vi "ImageFile_GetFolderImageFiles.vi"(8 "error in (no error)":errorcluster, 11 "File Path":path) -> (0 "error out":errorcluster, 3 "Folder Image Files":path[](array[path]))   [LabVIEW 2019]
panel:
  out "index of element":i32
  out "filenames":string[](array[string])
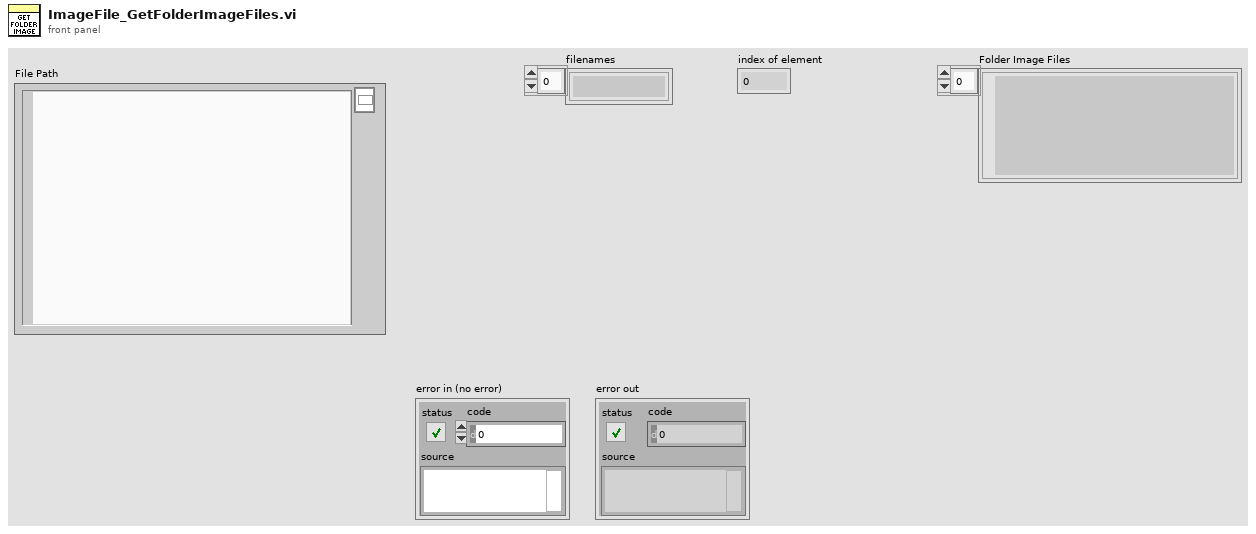
[diagram p1: front panel]
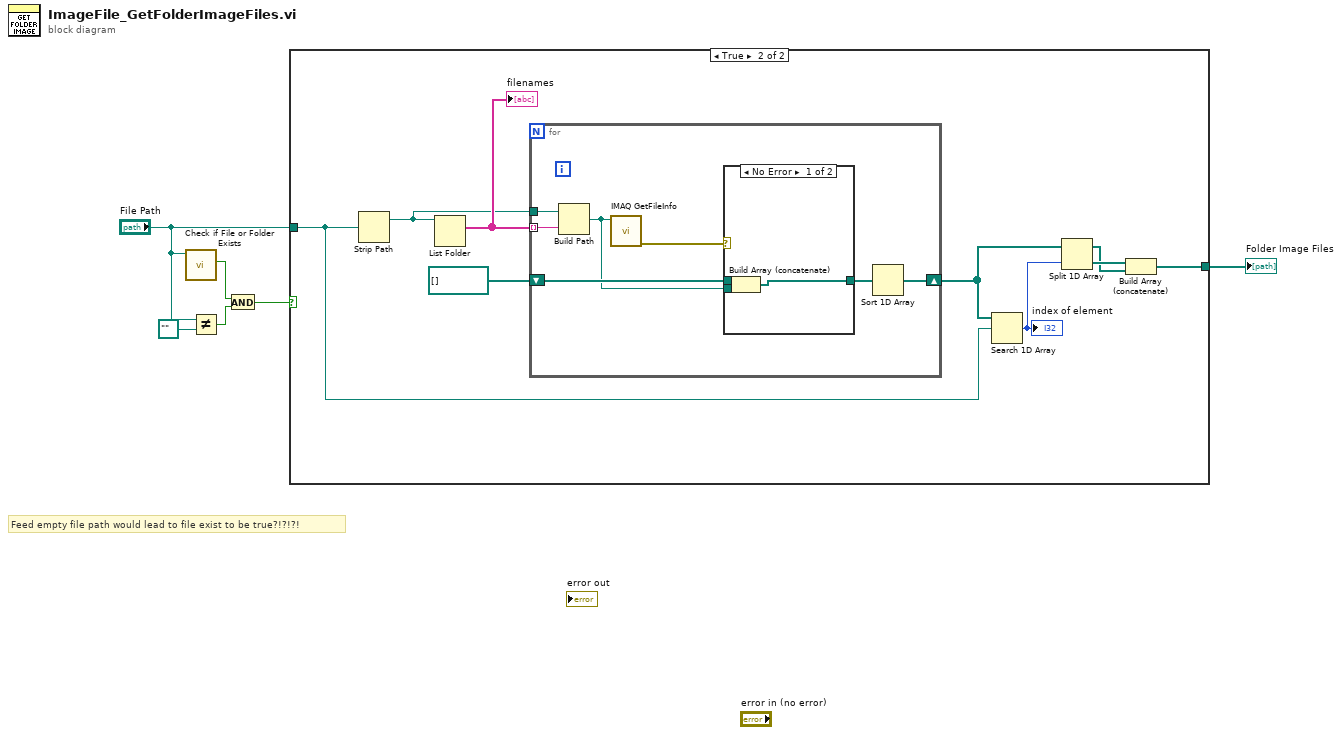
[diagram p0: block diagram]
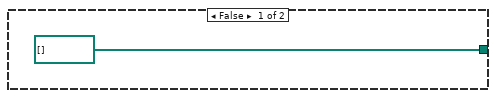
[diagram p2: hidden frame]
diagram:
  # "Feed empty file path would lead to file exist to be true?!?!?!"
  n1 = call <vilib>:"Check if File or Folder Exists.vi"("path"="File Path") -> ("file or folder exists?"=w2:bool)  [unwired: 8 in, 2 out]
  n2 = Not Equal?(x="File Path", y=path "") -> (x != y?=w3:bool)
  n3 = And(x=w2, y=w3) -> (x .and. y?=w1:bool)
  n4 = case shown="True" w1 {
    tunnel: [path[] [] w11] -> w6
    tunnel: "File Path" -> [_ w8]
    frame False {
    }
    frame True {
      n5 = Strip Path(path=w8) -> (stripped path=w15:path)  [unwired: 1 out]
      n6 = List Folder(path=w15) -> (filenames=w16:string[])  [unwired: 3 in, 3 out]
      "filenames" <- w16
      n7 = for {
        tunnel: w16 -> [w22] mode=indexing
        tunnel: w15 -> [w23]
        shift-right: [w17] -> w13
        shift-left: path[] [] -> [w20]
        n8 = Build Path(base path=w23, name or relative path=w22) -> (appended path=w19:path)
        n9 = call "IMAQ GetFileInfo"("File Path"=w19) -> ("error out"=w21:errorcluster)  [unwired: 4 in, 6 out]
        n10 = case shown="No Error" w21 {
          tunnel: w20 -> [w26 w27]
          tunnel: w19 -> [w25 _]
          tunnel: [w24 w27] -> w18
          frame No Error {
            n11 = Build Array (concatenate)(w26, w25) -> (w24:path[])
          }
          frame Error {
          }
        }
        n12 = Sort 1D Array(array=w18) -> (sorted array=w17:path[])
      }
      n13 = Search 1D Array(1D array=w13, element=w8) -> (index of element=w12:i32)  [unwired: 1 in]
      "index of element" <- w12
      n14 = Split 1D Array(array=w13, index=w12) -> (first subarray=w9:path[], second subarray=w10:path[])
      n15 = Build Array (concatenate)(w10, w9) -> (w11:path[])
    }
  }
  "Folder Image Files" <- w6
